vi "SR830_AutoSens.vi"(3 "Sensitivity":i32, 5 "Data in":dbl[](array[numeric])=[11.0, 222.0, 3.0, 4.0]) -> (0 "Sensitivity Out":i32, 1 "Set Sensitivity":bool=TRUE, 2 "Data out":dbl[](array[numeric]))   [LabVIEW 2019]
uses:
  Instrument_Setup.vi
panel:
  out "Numeric 2":dbl format="%#_13g"
  out "Numeric":dbl format="%#_13g"
  in  "Array":dbl[](array[numeric])=[2e-09, 5e-09, 1e-08, 2e-08, 5e-08, 1e-07, 2e-07, 5e-07, 1e-06, 2e-06, 5e-06, 1e-05, 2e-05, 5e-05, 0.0001, 0.0002, 0.0005, 0.001, 0.002, 0.005, 0.01, 0.02, 0.05, 0.1, 0.2, 0.5, 1.0]
  out "Decrease":bool=TRUE
  out "Increase":bool=TRUE
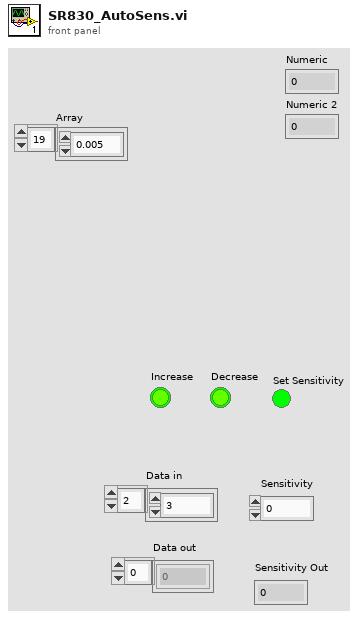
[diagram p1: front panel]
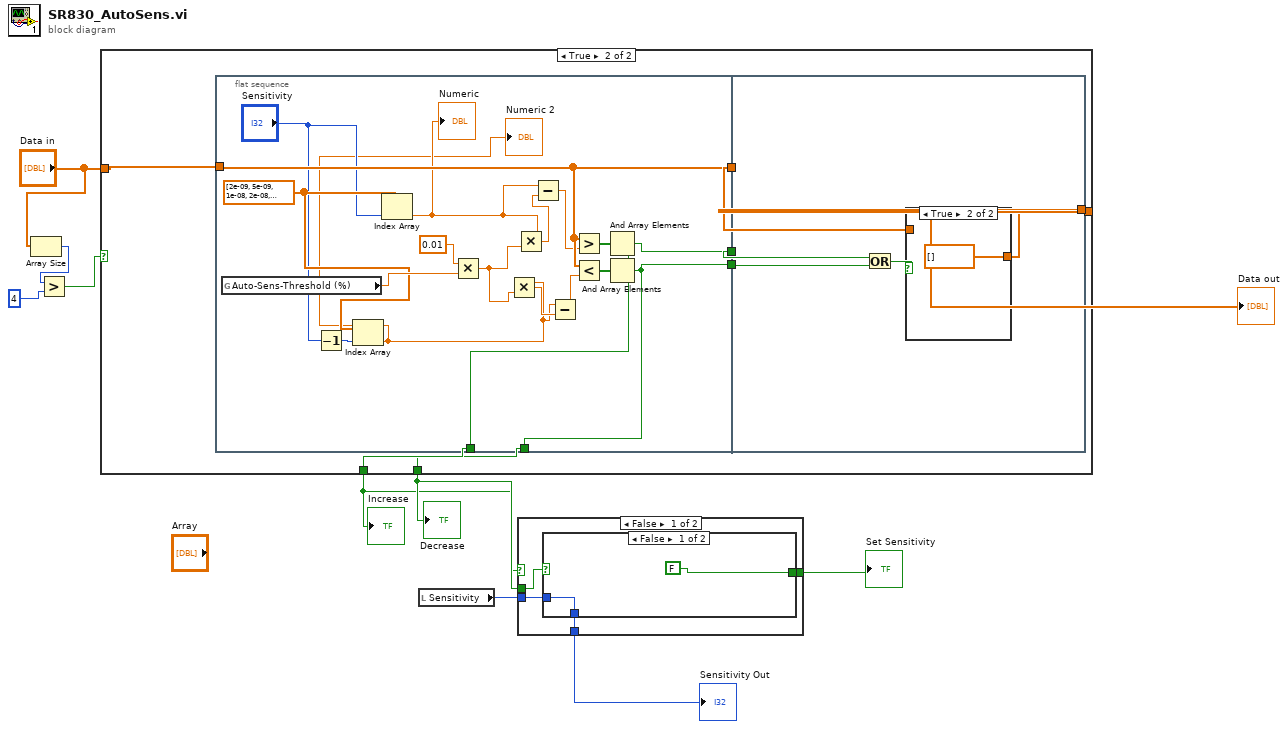
[diagram p0: block diagram]
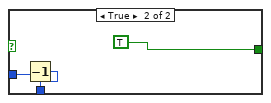
[diagram p2: hidden frame]
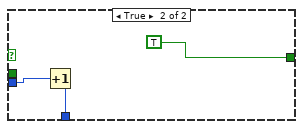
[diagram p3: hidden frame]
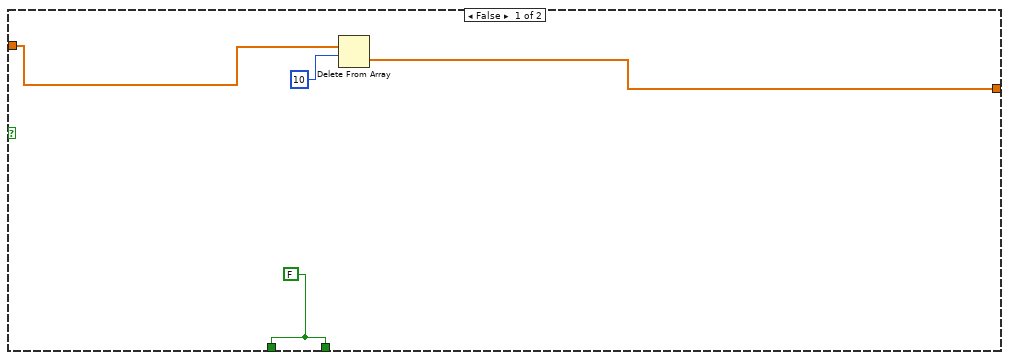
[diagram p4: hidden frame]
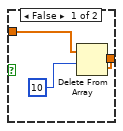
[diagram p5: hidden frame]
diagram:
  n1 = Array Size(array="Data in") -> (size(s)=w9:i32)
  n2 = Greater?(x=w9, y=4) -> (0:w8:bool)
  n3 = case shown="True" w8 {
    tunnel: "Data in" -> [w13 w21]
    tunnel: [w11 w18] -> w6
    tunnel: [w14 w16] -> w4
    tunnel: [w14 w15] -> w5
    frame False {
      w14 = FALSE
      n4 = Delete From Array(array=w13, length=10) -> (deleted portion=w11:dbl[])  [unwired: 1 in, 1 out]
    }
    frame True {
      n5 = flat-sequence {
        tunnel: w21 -> [w36]
        tunnel: [w35] -> w20
        tunnel: [w34] -> w19
        tunnel: [w36] -> w17
        tunnel: [w35] -> w16
        tunnel: [w34] -> w15
        tunnel: w20 -> [w43]
        tunnel: w19 -> [w42]
        tunnel: [w40] -> w18
        tunnel: w17 -> [w39]
        frame #0 {
          w31 = dbl[] [2e-09, 5e-09, 1e-08, 2e-08, 5e-08, 1e-07, 2e-07, 5e-07, 1e-06, 2e-06, 5e-06, 1e-05, 2e-05, 5e-05, 0.0001, 0.0002, 0.0005, 0.001, 0.002, 0.005, 0.01, 0.02, 0.05, 0.1, 0.2, 0.5, 1.0] ("Array")
          n6 = global read "Instrument_Setup.vi" "Auto-Sens-Threshold (%)"() -> (w33:dbl)
          n7 = Decrement(x="Sensitivity") -> (x-1=w30:i32)
          n8 = Index Array(array=w31, index=w30) -> (element=w24:dbl)
          "Numeric 2" <- w24
          n9 = Index Array(array=w31, index="Sensitivity") -> (element=w27:dbl)
          "Numeric" <- w27
          n10 = Multiply(x=0.01, y=w33) -> (x*y=w22:dbl)
          n11 = Multiply(x=w24, y=w22) -> (x*y=w25:dbl)
          n12 = Multiply(x=w27, y=w22) -> (x*y=w28:dbl)
          n13 = Subtract(x=w27, y=w28) -> (x-y=w26:dbl)
          n14 = Subtract(x=w24, y=w25) -> (x-y=w23:dbl)
          n15 = Greater?(x=w36, y=w26) -> (0:w38:bool[])
          n16 = Less?(x=w36, y=w23) -> (x < y?=w37:bool[])
          n17 = And Array Elements(Boolean array=w38) -> (logical AND=w35:bool)
          n18 = And Array Elements(Boolean array=w37) -> (logical AND=w34:bool)
        }
        frame #1 {
          n19 = Or(x=w43, y=w42) -> (x .or. y?=w41:bool)
          n20 = case shown="True" w41 {
            tunnel: [w44 dbl[] []] -> w40
            tunnel: w39 -> [w45 _]
            frame False {
              n21 = Delete From Array(array=w45, length=10) -> (deleted portion=w44:dbl[])  [unwired: 1 in, 1 out]
            }
            frame True {
            }
          }
        }
      }
    }
  }
  "Data out" <- w6
  "Decrease" <- w5
  "Increase" <- w4
  n22 = local read "Sensitivity"() -> (w3:i32)
  n23 = case shown="False" w4 {
    tunnel: w3 -> [w50 w59]
    tunnel: w5 -> [w51 _]
    tunnel: [w49 TRUE] -> w2
    tunnel: [w48 w57] -> w1
    frame False {
      n24 = case shown="False" w51 {
        tunnel: w50 -> [w52 w56]
        tunnel: [FALSE TRUE] -> w49
        tunnel: [w52 w54] -> w48
        frame False {
        }
        frame True {
          n25 = Decrement(x=w56) -> (x-1=w54:i32)
        }
      }
    }
    frame True {
      n26 = Increment(x=w59) -> (x+1=w57:i32)
    }
  }
  "Set Sensitivity" <- w2
  "Sensitivity Out" <- w1
